vi "CPU_MEM_VIC-II.vi"(5 "read all":bool, 7 "oper":enum16{"init", "read", "write"}(ring), 10 "value in":u8 format="%02x", 11 "address":u16 format="%04x") -> (2 "value out":u8 format="%02x", 3 "mem":u8[](array[numeric]) format="%02x")   [LabVIEW 2018]
uses:
  VIC/VIC_IRQ_oper.ctl
  VIC/VIC_glb.vi
panel:
  in  "init size":u16=1023 format="%.0x"
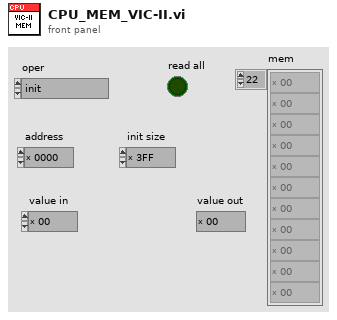
[diagram p1: front panel]
types:
  T1 = typedef "VIC_IRQ_oper.ctl" = enum16{"init", "set mask", "set flag", "check active", "read reg", "reset flag"}
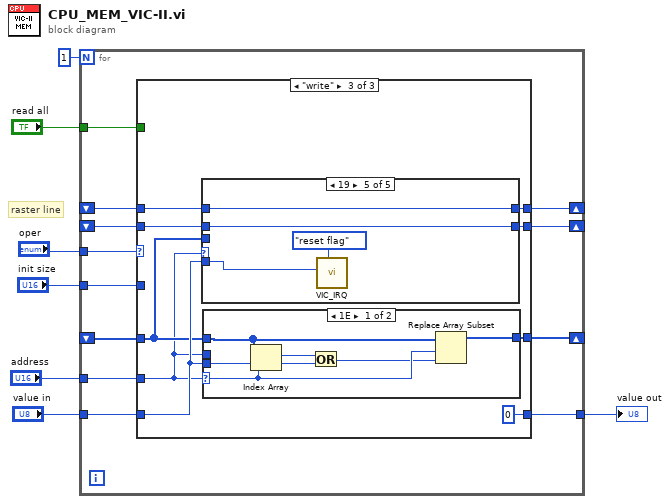
[diagram p0: block diagram]
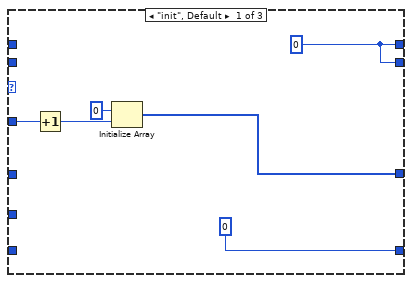
[diagram p2: hidden frame]
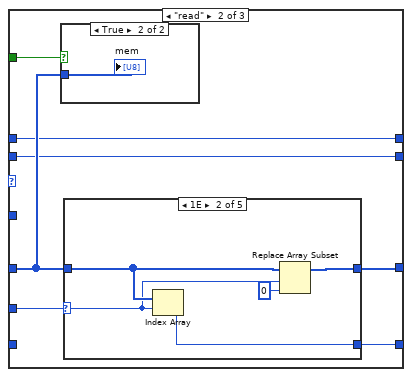
[diagram p3: hidden frame]
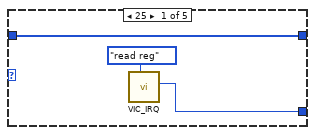
[diagram p5: hidden frame]
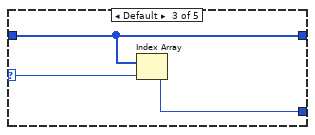
[diagram p6: hidden frame]
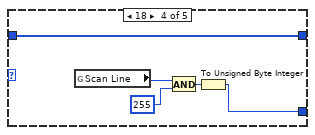
[diagram p7: hidden frame]
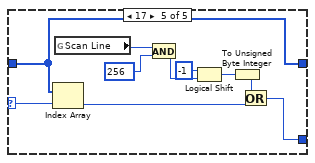
[diagram p8: hidden frame]
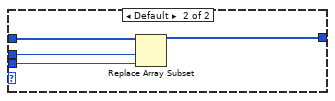
[diagram p9: hidden frame]
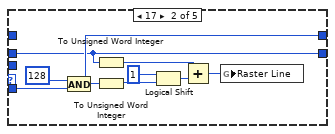
[diagram p11: hidden frame]
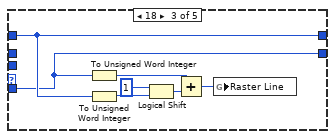
[diagram p12: hidden frame]
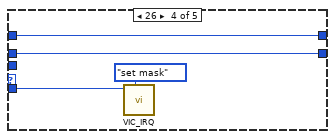
[diagram p13: hidden frame]
diagram:
  # "raster line"
  n1 = for {
    N: 1 -> [_]
    shift-right: [w17] -> _
    shift-left: _ -> [w16]
    tunnel: "oper" -> [w19]
    tunnel: "init size" -> [w18]
    tunnel: [w15] -> w4
    tunnel: "address" -> [w14]
    tunnel: "value in" -> [w13]
    tunnel: "read all" -> [w12]
    shift-right: [w11] -> _
    shift-left: _ -> [w9]
    shift-right: [w10] -> _
    shift-left: _ -> [w8]
    n2 = case shown="\"write\"" w19 {
      tunnel: w18 -> [w25 _ _]
      tunnel: [w23 w26 w68] -> w17
      tunnel: w16 -> [_ w30 w61]
      tunnel: [u8 0 ("element") w32 u8 0 ("element")] -> w15
      tunnel: w14 -> [_ w31 w60]
      tunnel: w13 -> [_ _ w66]
      tunnel: w12 -> [_ w29 _]
      tunnel: [w20 w27 w65] -> w11
      tunnel: [w20 w28 w64] -> w10
      tunnel: w9 -> [_ w27 w63]
      tunnel: w8 -> [_ w28 w62]
      frame "init", Default {
        w20 = u8 0
        n3 = Increment(x=w25) -> (x+1=w21:u16)
        n4 = Initialize Array(u8 0 ("element"), w21) -> (w23:u8[])
      }
      frame "read" {
        n5 = case shown="True" w29 {
          tunnel: w30 -> [_ w33]
          frame False {
          }
          frame True {
            "mem" <- w33
          }
        }
        n6 = case shown="1E" w31 {
          selector: w31 -> [_ w38 w43 _ w55]
          tunnel: w30 -> [w34 w39 w42 w45 w50]
          tunnel: [w36 w41 w44 w46 w51] -> w32
          tunnel: [w34 w40 w42 w45 w50] -> w26
          frame 25 {
            n7 = call "VIC_IRQ.vi"("oper"=VIC_IRQ_oper."read reg") -> ("IRQ.reg"=w36:u8)  [unwired: 8 in, 2 out]
          }
          frame 30 {
            n8 = Index Array(array=w39, index=w38) -> (element=w41:u8)
            n9 = Replace Array Subset(array=w39, new element=u8 0 ("new element/subarray"), index=w38) -> (w40:u8[])
          }
          frame Default {
            n10 = Index Array(array=w42, index=w43) -> (element=w44:u8)
          }
          frame 18 {
            n11 = global read "VIC_glb.vi" "Scan Line"() -> (w49:u16)
            n12 = And(x=w49, y=u16 255) -> (x .and. y?=w47:u16)
            n13 = To Unsigned Byte Integer(number=w47) -> (unsigned 8bit integer=w46:u8)
          }
          frame 17 {
            n14 = Index Array(array=w50, index=w55) -> (element=w54:u8)
            n15 = global read "VIC_glb.vi" "Scan Line"() -> (w59:u16)
            n16 = And(x=w59, y=u16 256) -> (x .and. y?=w56:u16)
            n17 = Logical Shift(y=i16 -1, x=w56) -> (x << y=w53:u16)
            n18 = To Unsigned Byte Integer(number=w53) -> (unsigned 8bit integer=w52:u8)
            n19 = Or(x=w52, y=w54) -> (x .or. y?=w51:u8)
          }
        }
      }
      frame "write" {
        n20 = case shown="19" w60 {
          tunnel: w66 -> [_ w88 w90 w100 w104]
          tunnel: [w79 w83 w90 w97 w101] -> w65
          tunnel: [w80 w86 w91 w98 w102] -> w64
          tunnel: w63 -> [w79 w83 _ w97 w101]
          tunnel: w62 -> [w80 _ w91 w98 w102]
          tunnel: w61 -> [_ _ _ _ _]
          frame Default {
          }
          frame 17 {
            n21 = And(x=u8 128 ("y"), y=w88) -> (x .and. y?=w86:u8)
            n22 = To Unsigned Word Integer(number=w83) -> (unsigned 16bit integer=w82:u16)
            n23 = To Unsigned Word Integer(number=w86) -> (unsigned 16bit integer=w84:u16)
            n24 = Logical Shift(y=i16 1, x=w84) -> (x << y=w85:u16)
            n25 = Add(x=w82, y=w85) -> (x+y=w81:u16)
            n26 = global write "VIC_glb.vi" "Raster Line"(w81) -> ()
          }
          frame 18 {
            n27 = To Unsigned Word Integer(number=w90) -> (unsigned 16bit integer=w93:u16)
            n28 = To Unsigned Word Integer(number=w91) -> (unsigned 16bit integer=w94:u16)
            n29 = Logical Shift(y=i16 1, x=w94) -> (x << y=w95:u16)
            n30 = Add(x=w93, y=w95) -> (x+y=w92:u16)
            n31 = global write "VIC_glb.vi" "Raster Line"(w92) -> ()
          }
          frame 26 {
            n32 = call "VIC_IRQ.vi"("oper"=VIC_IRQ_oper."set mask", "mask value"=w100) -> ()  [unwired: 7 in, 3 out]
          }
          frame 25 {
            n33 = call "VIC_IRQ.vi"("oper"=VIC_IRQ_oper."reset flag", "IRQ flag idx"=w104) -> ()  [unwired: 7 in, 3 out]
          }
        }
        n34 = case shown="1E" w60 {
          selector: w60 -> [w72 _]
          tunnel: [w74 w78] -> w68
          tunnel: w60 -> [_ w77]
          tunnel: w66 -> [w70 w76]
          tunnel: w61 -> [w73 w75]
          frame 30 {
            n35 = Index Array(array=w73, index=w72) -> (element=w71:u8)
            n36 = Or(x=w71, y=w70) -> (x .or. y?=w69:u8)
            n37 = Replace Array Subset(array=w73, new element=w69, index=w72) -> (w74:u8[])
          }
          frame Default {
            n38 = Replace Array Subset(array=w75, new element=w76, index=w77) -> (w78:u8[])
          }
        }
      }
    }
  }
  "value out" <- w4
